vi "render.vi"(11 "ArrayIn":bool[][](array[boolean])) -> (2 "pictureOut":picture)   [LabVIEW 2021]
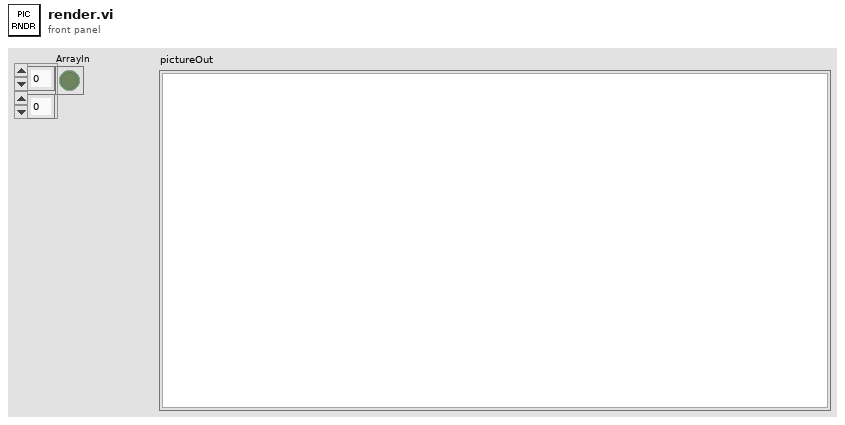
[diagram p1: front panel]
types:
  T1 = typedef "imagedata.ctl" = cluster{"image type":i32, "image depth":i32, "image":u8[], "mask":u8[], "colors":u32[], "Rectangle":cluster{"left":i16, "top":i16, "right":i16, "bottom":i16}}
  T2 = cluster{"line color":u32, "text color":u32, "tick length":i16, "crossing axes":bool, "visible grid?":bool}
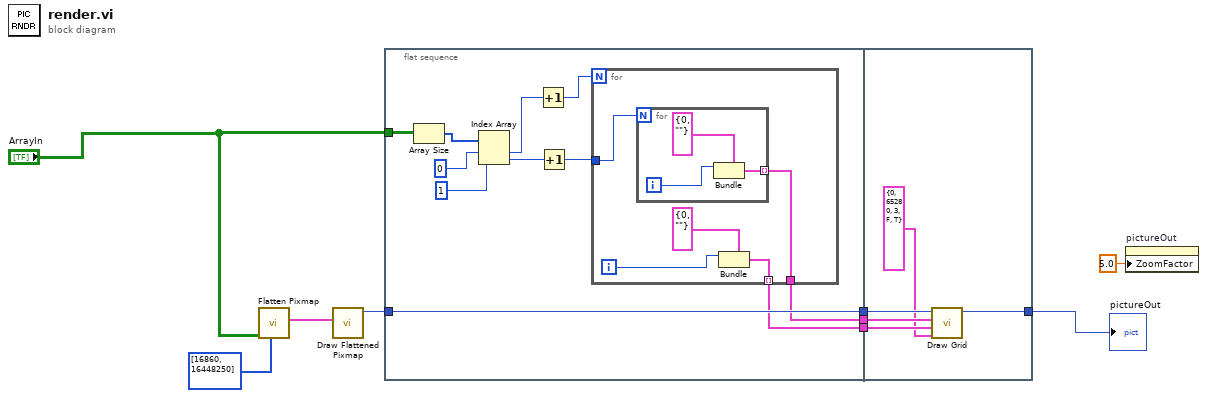
[diagram p0: block diagram]
diagram:
  n1 = call <vilib>:"Flatten Pixmap.vi"("colors"=u32[] [16860, 16448250], "1-bit pixmap"="ArrayIn") -> ("image data"=w6:T1)  [unwired: 9 in]
  n2 = call <vilib>:"Draw Flattened Pixmap.vi"("image data"=w6) -> ("new picture"=w4:picture)  [unwired: 8 in]
  n3 = flat-sequence {
    tunnel: w4 -> [w20]
    tunnel: [w20] -> w9
    tunnel: [w16] -> w8
    tunnel: [w15] -> w7
    tunnel: "ArrayIn" -> [w14]
    tunnel: [w32] -> w3
    tunnel: w9 -> [w33]
    tunnel: w8 -> [w31]
    tunnel: w7 -> [w30]
    frame #0 {
      n4 = Array Size(array=w14) -> (size(s)=w19:i32[])
      n5 = Index Array(array=w19, index #1=0 ("index"), index #2=1 ("index")) -> (element #1=w13:i32, element #2=w10:i32)
      n6 = Increment(x=w13) -> (x+1=w12:i32)
      n7 = Increment(x=w10) -> (x+1=w11:i32)
      n8 = for {
        N: w12 -> [_]
        tunnel: [w24] -> w15 mode=indexing
        tunnel: [w23] -> w16
        tunnel: w11 -> [w22]
        i -> [w21]
        n9 = for {
          N: w22 -> [_]
          tunnel: [w27] -> w23 mode=indexing
          i -> [w26]
          n10 = Bundle(cluster=cluster{"coordinate":i32, "label":string} {"coordinate"=0, "label"=""} ("decade specs"), "coordinate"=w26) -> (w27:cluster{"coordinate":i32, "label":string})  [unwired: 1 in]
        }
        n11 = Bundle(cluster=cluster{"coordinate":i32, "label":string} {"coordinate"=0, "label"=""} ("decade specs"), "coordinate"=w21) -> (w24:cluster{"coordinate":i32, "label":string})  [unwired: 1 in]
      }
    }
    frame #1 {
      n12 = call <vilib>:"Draw Grid.vi"("grid cosmetics"=T2 {"line color"=0, "text color"=65280, "tick length"=3, "crossing axes"=FALSE, "visible grid?"=TRUE}, "y scale specs"=w30, "x scale specs"=w31, "picture"=w33) -> ("new picture"=w32:picture)  [unwired: 5 in]
    }
  }
  n13 = property on="pictureOut" class="Pict"("ZoomFactor"=sgl 5.0 ("Zoom Factor")) -> ()  [unwired: 2 in, 2 out]
  "pictureOut" <- w3
